vi "GetPowerE4418b.vi"(2 "error in (no error)":errorcluster) -> (0 "Error out":errorcluster, 1 "Power returned (dBm)":dbl format="%#.10f")   [LabVIEW 2009]
doc: "Gets a power reading from the E4418B power meter."
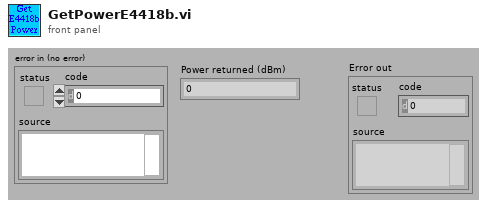
[diagram p1: front panel]
types:
  T1 = enum16{"N1911A", "Siggen", "34980a", "E4418B", "Rvp8"}
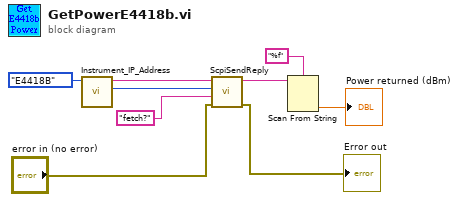
[diagram p0: block diagram]
diagram:
  n1 = call "Instrument_IP_Address.vi"("Instrument"=T1."E4418B") -> ("Port"=w1:u16, "IP Address"=w2:string)  [unwired: 9 in]
  n2 = call "ScpiSendReply.vi"("error in (no error)"="error in (no error)", "Command"="fetch?" ("format string"), "TCP port"=w1, "IP Address"=w2) -> ("Error out"=→"Error out":errorcluster, "Reply"=w7:string)  [unwired: 5 in]
  n3 = Scan From String(format string="%f", input string=w7) -> (output 1=→"Power returned (dBm)":dbl)  [unwired: 3 in, 3 out]
